vi "Main.vi"() -> ()   [LabVIEW 2020]
uses:
  <vilib>/vision/NI_Vision_Development_Module.lvlib
panel:
  out "Image":T1(plugin-control)
  in  "停止":bool
  out "error out":errorcluster
  out "Number of Objects":i32
  in  "Settings":T2={"Objects"=0, "Threshold"=128, "Reject Border"=FALSE, "Fill Holes"=FALSE, "Min Object Size"=FALSE, "Min Size"=3, "Max Object Size"=FALSE, "Max Size"=100, "Show Search Area"=FALSE, "Show Center"=TRUE, "Show Bounding Box"=TRUE} {"Objects" items=["Bright Objects", "Dark Objects"]; "Threshold" min=1 max=999999999 step=1; "Max Size" min=1 max=999999999 step=1; "Min Size" min=1 max=999999999 step=1}
  in  "File Path":path
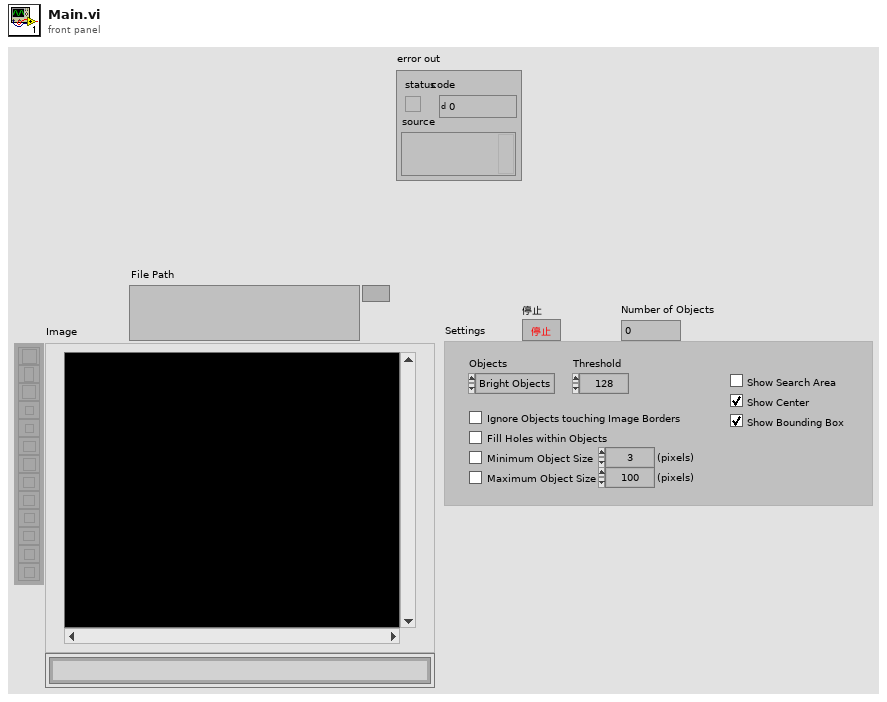
[diagram p1: front panel]
types:
  T1 = typedef "IMAQ Image.ctl" = refnum<image>
  T2 = cluster{"Objects":u16, "Threshold":i32, "Reject Border":bool, "Fill Holes":bool, "Min Object Size":bool, "Min Size":i32, "Max Object Size":bool, "Max Size":i32, "Show Search Area":bool, "Show Center":bool, "Show Bounding Box":bool}
  T3 = typedef "Image Type" = u32
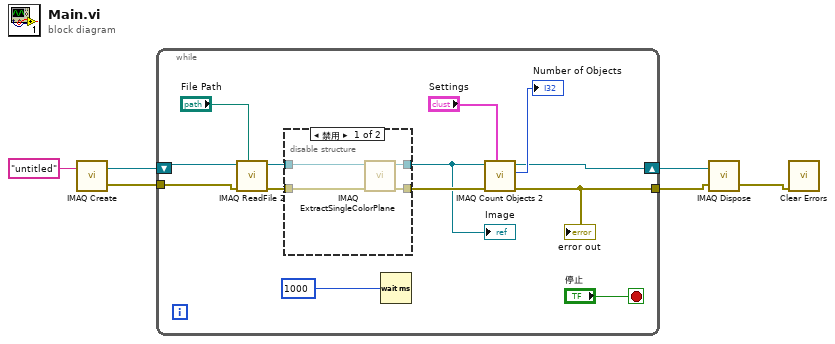
[diagram p0: block diagram]
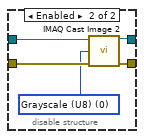
[diagram p2: hidden frame]
diagram:
  n1 = call "IMAQ Create"("Image Name"="untitled") -> ("New Image"=w5:T1, "error out"=w4:errorcluster)  [unwired: 4 in]
  n2 = while {
    tunnel: w4 -> [w17]
    shift-right: [w11] -> w3
    shift-left: w5 -> [w18]
    tunnel: [w10] -> w2
    stop <- "停止" stop-if-true
    n3 = call "IMAQ ReadFile 2"("File Path"="File Path", "error in (no error)"=w17, "Image"=w18) -> ("error out"=w15:errorcluster, "Image Out"=w16:T1)  [unwired: 4 in, 3 out]
    n4 = disable-structure shown="禁用" {
      disable-tunnel: w16 -> [w23 w28]
      disable-tunnel: w15 -> [w22 w27]
      disable-tunnel: [w21 w26] -> w12
      disable-tunnel: [w20 w25] -> w7
      frame Disabled {
        n5 = call "IMAQ ExtractSingleColorPlane"("error in (no error)"=w22, "Image Src"=w23) -> ("error out"=w21:errorcluster, "Image Dst Out"=w20:T1)  [unwired: 8 in]
      }
      frame Enabled {
        w24 = T3 0 items=["Grayscale (U8)", "Grayscale (I16)", "Grayscale (SGL)", "Complex (CSG)", "RGB (U32)", "HSL (U32)", "RGB (U64)", "Grayscale (U16)"] ("Image Type")
        n6 = call "IMAQ Cast Image 2"("Image Src"=w28, "Image Type"=w24, "error in (no error)"=w27) -> ("Image Dst Out"=w25:T1, "error out"=w26:errorcluster)  [unwired: 11 in]
      }
    }
    "Image" <- w7
    n7 = Wait (ms)(milliseconds to wait=u32 1000 ("等待时间（毫秒）")) -> ()  [unwired: 1 out]
    n8 = call "IMAQ Count Objects 2"("Settings"="Settings", "error in (no error)"=w12, "Image"=w7) -> ("error out"=w10:errorcluster, "Number of Objects"=→"Number of Objects":i32, "Image Out"=w11:T1)  [unwired: 4 in, 2 out]
    "error out" <- w10
  }
  n9 = call "IMAQ Dispose"("Image"=w3, "error in (no error)"=w2) -> ("error out"=w1:errorcluster)  [unwired: 4 in]
  n10 = call <vilib>:"Clear Errors.vi"("error in (no error)"=w1) -> ()  [unwired: 5 in, 2 out]
